vi "test.vi"() -> ()   [LabVIEW 2015]
uses:
  <vilib>/Analysis/6fits.llb/Curve Fitting Criteria.ctl
  APP/subject_class/elabPhases.ctl
  <userlib>/Read_Excel_Values.llb/GetXL_CellValues_2D_String.vi
  <vilib>/Analysis/NI_AALPro.lvlib
  APP/subject_class/subject.lvclass
panel:
  out "Array":i32[](array[numeric])
  out "XY Graph 3":cluster{i32[], "Best Linear Fit":dbl[]}[](graph)
  in  "Stop Button":bool
  out "XY Graph 2":cluster{"Best Linear Fit":dbl[], dbl[]}[](graph)
  out "output array":string[][](array[string])
  out "Array 3":i32[](array[numeric])
  out "Array 2":string[](array[string])
  in  "path":path
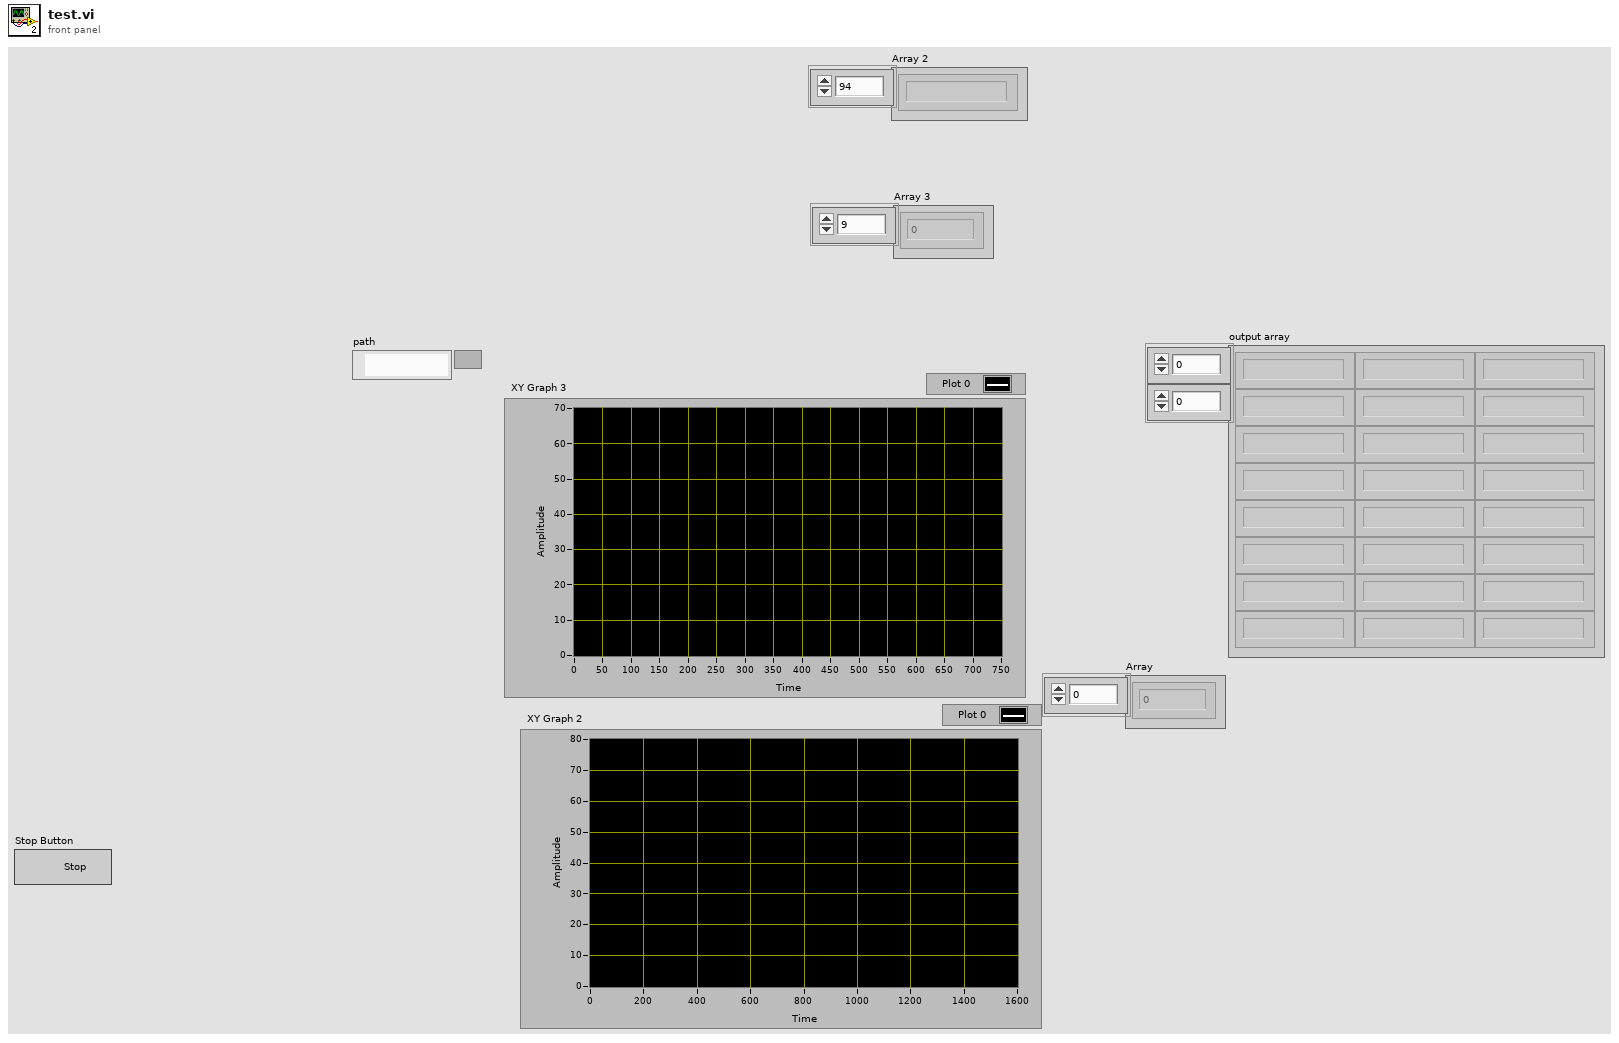
[diagram p1: front panel]
types:
  T1 = typedef "subject.lvclass/elabPhases.ctl" = enum16{"over", "under", "intersec"}
  T2 = typedef "NI_AALPro.lvlib/Curve Fitting Criteria.ctl" = u16
  T3 = cluster{"Excel._Application":refnum<k7>, "Workbooks":refnum<k7>}
  T4 = cluster{"Excel._Application":refnum<k7>, "Workbooks":refnum<k7>, "Open":refnum<k7>}
  T5 = cluster{"Excel._Application":refnum<k7>, "Workbooks":refnum<k7>, "Open":refnum<k7>, "Worksheets":refnum<k7>, "Excel._Worksheet":refnum<k7>}
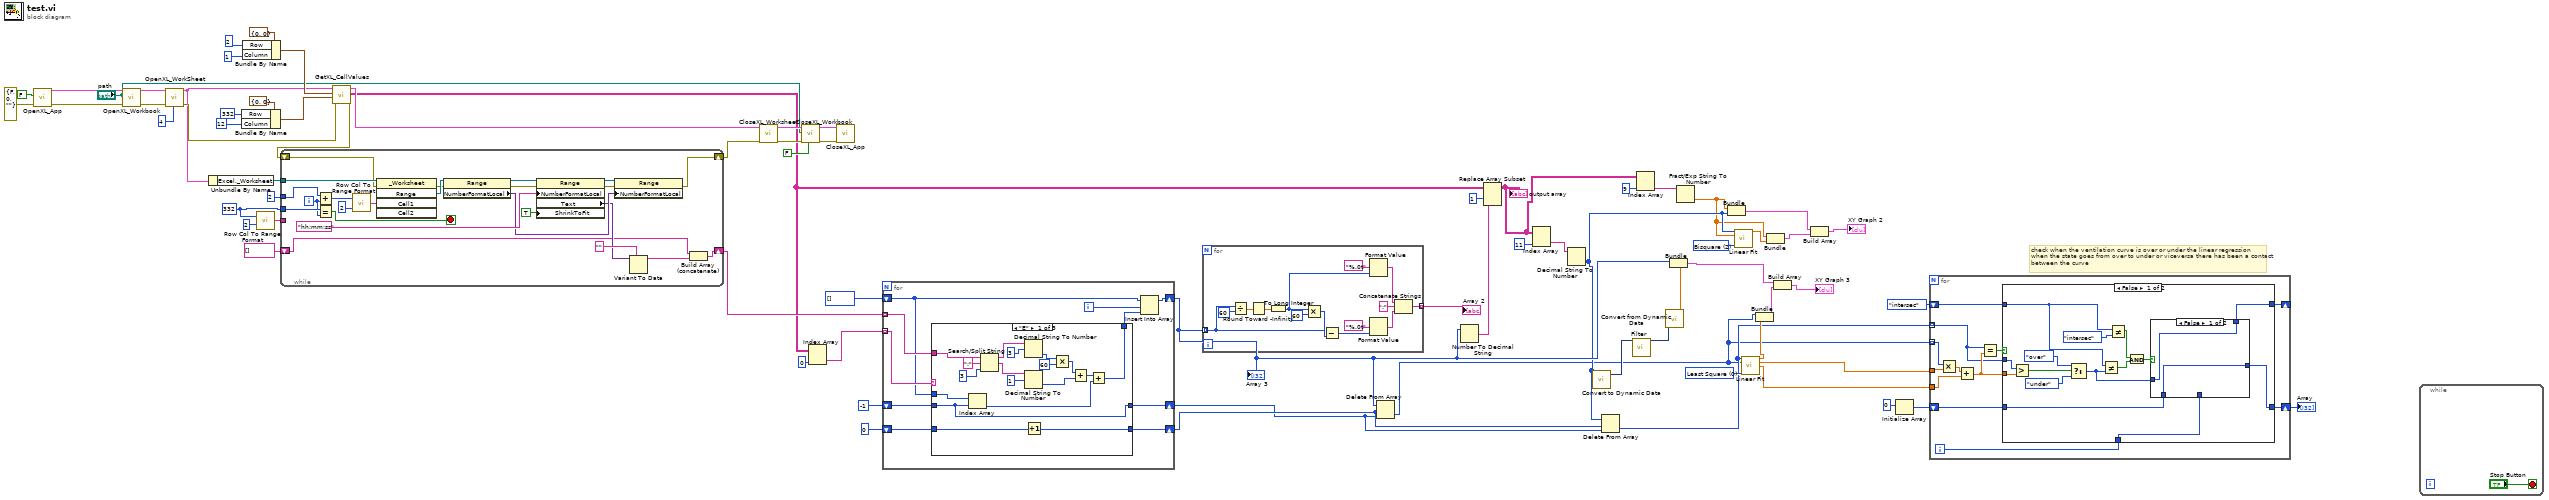
[diagram p0: block diagram]
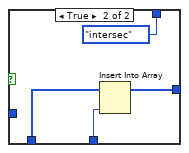
[diagram p2: hidden frame]
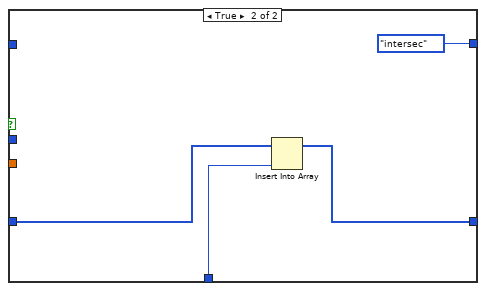
[diagram p3: hidden frame]
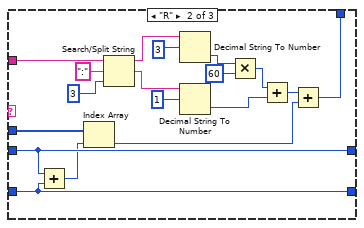
[diagram p4: hidden frame]
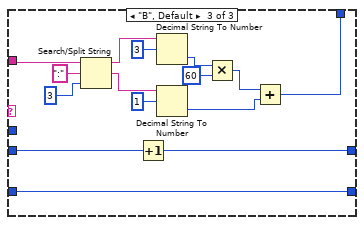
[diagram p5: hidden frame]
diagram:
  w9 = T2 2 items=["Least Square", "Least Absolute Residual", "Bisquare"] ("method")
  w32 = T2 0 items=["Least Square", "Least Absolute Residual", "Bisquare"] ("method")
  w42 = 332 ("Column")
  # "check when the ventilation curve is over or under the linear regression\nwhen the state goes from over to under or viceversa there has been a contact\nbetween the curve"
  n1 = call <userlib>:"OpenXL_App.vi"("error in (no error)"=errorcluster {"status"=FALSE, "code"=0, "source"=""}, "Visible"=FALSE) -> ("error out"=w66:errorcluster, "Refnum Cluster"=w67:T3)  [unwired: 8 in]
  n2 = call <userlib>:"OpenXL_Workbook.vi"("error in"=w66, "path"="path", "Refnum Cluster In"=w67) -> ("error out"=w65:errorcluster, "Refnum Cluster Out"=w47:T4)  [unwired: 7 in]
  n3 = call <userlib>:"OpenXL_WorkSheet.vi"("Sheet"=4, "error in (no error)"=w65, "Refnum Cluster In"=w47) -> ("error out"=w57:errorcluster, "Refnum Cluster Out"=w37:T5)  [unwired: 7 in]
  n4 = Unbundle By Name(w37) -> ("Excel._Worksheet"=w46:refnum<k7>)
  n5 = Bundle By Name(cluster=cluster{"Column":i32, "Row":i32} {"Column"=0, "Row"=0} ("Start"), "Row"=332, "Column"=12) -> (w58:cluster{"Column":i32, "Row":i32})
  n6 = Bundle By Name(cluster=cluster{"Column":i32, "Row":i32} {"Column"=0, "Row"=0} ("Start"), "Row"=2 ("Column"), "Column"=1) -> (w59:cluster{"Column":i32, "Row":i32})
  n7 = call <userlib>:"Row Col To Range Format.vi"("Column"=2, "Row"=w42) -> ("Output String"=w44:string)
  n8 = call-poly <userlib>:"GetXL_CellValues.vi"("error in"=w57, "End"=w58, "Start"=w59, "Refnum Cluster In"=w37) -> ("error out"=w40:errorcluster, "data"=w20:string[][], "Refnum Cluster Out"=w54:T5)  [unwired: 5 in]
  n9 = while {
    tunnel: w46 -> [w91]
    tunnel: w44 -> [_]
    shift-right: [w84] -> w38
    shift-left: string[] [] -> [w86]
    tunnel: w42 -> [w83]
    tunnel: 2 ("Column") -> [w79]
    shift-right: [w75] -> w39
    shift-left: w40 -> [w74]
    i -> [w78]
    stop <- w82 stop-if-true
    n10 = Add(x=w79, y=w78) -> (x+y=w77:i32)
    n11 = Equal?(x=w83, y=w78) -> (x = y?=w82:bool)
    n12 = call <userlib>:"Row Col To Range Format.vi"("Column"=2, "Row"=w77) -> ("Output String"=w80:string)
    n13 = invoke class="_Worksheet" method="Range"(reference=w91, error in=w74, "Cell1"=w80) -> (error out=w95:errorcluster, "Range"=w97:refnum<k7>)  [unwired: 2 in, 3 out]
    n14 = property class="Range"(reference=w97, error in=w95) -> (reference out=w96:refnum<k7>, error out=w94:errorcluster, "NumberFormatLocal"=w92:variant)
    n15 = property class="Range"(reference=w96, error in=w94, "NumberFormatLocal"="hh:mm:ss" ("data 3"), "ShrinkToFit"=TRUE) -> (reference out=w88:refnum<k7>, error out=w76:errorcluster, "Text"=w89:variant)
    n16 = property class="Range"(reference=w88, error in=w76, "NumberFormatLocal"=w92) -> (error out=w75:errorcluster)  [unwired: 1 out]
    n17 = Variant To Data(type="", Variant=w89) -> (data=w85:string)  [unwired: 1 in, 1 out]
    n18 = Build Array (concatenate)(w86, w85) -> (w84:string[])
  }
  n19 = call <userlib>:"CloseXL_Worksheet.vi"("error in (no error)"=w39, "Refnum Cluster In"=w54) -> ("error out"=w51:errorcluster, "Refnum Cluster Out"=w52:T4)  [unwired: 8 in]
  n20 = call <userlib>:"CloseXL_Workbook.vi"("Save? (F)"=FALSE, "error in (no error)"=w51, "path"="path", "Refnum Cluster In"=w52) -> ("error out"=w49:errorcluster, "Refnum Cluster Out"=w50:T3)  [unwired: 6 in]
  n21 = Index Array(array=w20, index (col)=0 ("disabled index (col)")) -> (element=w71:string[])  [unwired: 1 in]
  n22 = call <userlib>:"CloseXL_App.vi"("error in (no error)"=w49, "Refnum Cluster In"=w50) -> ()  [unwired: 9 in, 1 out]
  n23 = for {
    tunnel: w38 -> [w106] mode=indexing
    shift-right: [w105] -> w18
    shift-left: i32[] [] -> [w101]
    tunnel: w71 -> [w107] mode=indexing
    shift-right: [w102] -> w28
    shift-left: -1 -> [w99]
    shift-right: [w100] -> w29
    shift-left: 0 -> [w98]
    i -> [w104]
    n24 = case shown="\"E\"" w107 {
      tunnel: w106 -> [w117 w132 w158]
      tunnel: [w111 w131 w149] -> w103
      tunnel: w99 -> [w108 w127 w148]
      tunnel: [w108 w127 w147] -> w102
      tunnel: w101 -> [w115 w133 _]
      tunnel: w98 -> [w113 w128 w146]
      tunnel: [w112 w128 w146] -> w100
      frame "E" {
        n25 = Index Array(array=w115, index=w108) -> (element=w114:i32)
        n26 = Search/Split String(string=w117, search string/char (-)=":", offset (0)=3) -> (substring before match=w123:string, match + rest of string=w122:string)  [unwired: 1 out]
        n27 = Decimal String To Number(string=w123, offset=3) -> (number=w121:i32)  [unwired: 1 in, 1 out]
        n28 = Decimal String To Number(string=w122, offset=1) -> (number=w118:i32)  [unwired: 1 in, 1 out]
        n29 = Increment(x=w113) -> (x+1=w112:i32)
        n30 = Multiply(x=w121, y=60) -> (x*y=w119:i32)
        n31 = Add(x=w119, y=w118) -> (x+y=w116:i32)
        n32 = Add(x=w116, y=w114) -> (x+y=w111:i32)
      }
      frame "R" {
        n33 = Add(x=w127, y=w128) -> (x+y=w126:i32)
        n34 = Index Array(array=w133, index=w126) -> (element=w134:i32)
        n35 = Search/Split String(string=w132, search string/char (-)=":", offset (0)=3) -> (substring before match=w141:string, match + rest of string=w140:string)  [unwired: 1 out]
        n36 = Decimal String To Number(string=w141, offset=3) -> (number=w139:i32)  [unwired: 1 in, 1 out]
        n37 = Decimal String To Number(string=w140, offset=1) -> (number=w136:i32)  [unwired: 1 in, 1 out]
        n38 = Multiply(x=w139, y=60) -> (x*y=w137:i32)
        n39 = Add(x=w137, y=w136) -> (x+y=w135:i32)
        n40 = Add(x=w135, y=w134) -> (x+y=w131:i32)
      }
      frame "B", Default {
        n41 = Search/Split String(string=w158, search string/char (-)=":", offset (0)=3) -> (substring before match=w155:string, match + rest of string=w154:string)  [unwired: 1 out]
        n42 = Increment(x=w148) -> (x+1=w147:i32)
        n43 = Decimal String To Number(string=w155, offset=3) -> (number=w153:i32)  [unwired: 1 in, 1 out]
        n44 = Decimal String To Number(string=w154, offset=1) -> (number=w150:i32)  [unwired: 1 in, 1 out]
        n45 = Multiply(x=w153, y=60) -> (x*y=w151:i32)
        n46 = Add(x=w151, y=w150) -> (x+y=w149:i32)
      }
    }
    n47 = Insert Into Array(array=w101, index=w104, new element=w103) -> (w105:i32[])
  }
  "Array 3" <- w18
  n48 = for {
    tunnel: w18 -> [w168] mode=indexing
    tunnel: [w167] -> w13 mode=indexing
    n49 = Divide(x=w168, y=60) -> (x/y=w166:dbl)
    n50 = Round Toward -Infinity(1:w166) -> (0:w165:dbl)
    n51 = To Long Integer(number=w165) -> (32bit integer=w161:i32)
    n52 = Multiply(x=w161, y=60) -> (x*y=w169:i32)
    n53 = Subtract(x=w168, y=w169) -> (x-y=w163:i32)
    n54 = Format Value(format string="%.0t", value (0)=w161) -> (output string=w162:string)  [unwired: 1 in]
    n55 = Format Value(format string="%.0t", value (0)=w163) -> (output string=w159:string)  [unwired: 1 in]
    n56 = Concatenate Strings(w162, ":" ("string"), w159) -> (w167:string)
  }
  "Array 2" <- w13
  n57 = Delete From Array(array=w18, length=w29, index=w28) -> (deleted portion=w5:i32[])  [unwired: 1 out]
  n58 = Number To Decimal String(number=w18) -> (decimal integer string=w17:string[])  [unwired: 1 in]
  n59 = Replace Array Subset(array=w20, new element=w17, index (col)=1 ("disabled index (col)")) -> (w26:string[][])  [unwired: 1 in]
  "output array" <- w26
  n60 = Index Array(array=w26, index (col)=11 ("index (row)")) -> (element=w35:string[])  [unwired: 1 in]
  n61 = Decimal String To Number(string=w35) -> (number=w11:i32[])  [unwired: 2 in, 1 out]
  n62 = call "Convert to Dynamic Data"("Array"=w11) -> ("Dynamic Data Type"=w34:dynamicdata)  [unwired: 3 in]
  n63 = Delete From Array(array=w11, length=w29, index=w28) -> (deleted portion=w6:i32[])  [unwired: 1 out]
  n64 = call "Filter"("Signal"=w34) -> ("Filtered Signal"=w33:dynamicdata)  [unwired: 9 in, 1 out]
  n65 = Index Array(array=w26, index (col)=9 ("index (row)")) -> (element=w25:string[])  [unwired: 1 in]
  n66 = call "Convert from Dynamic Data"("Dynamic Data Type"=w33) -> ("Array"=w12:dbl[])  [unwired: 3 in]
  n67 = Bundle(w18, "Array"=w12) -> (w31:cluster{i32[], "Array":dbl[]})  [unwired: 1 in]
  n68 = Fract/Exp String To Number(string=w25) -> (number=w10:dbl[])  [unwired: 3 in, 1 out]
  n69 = Bundle(w10, w11) -> (w24:cluster{dbl[], i32[]})  [unwired: 1 in]
  n70 = call <vilib>:"Linear Fit.vi"("Y"=w11, "X"=w10, "method"=w9) -> ("Best Linear Fit"=w22:dbl[])  [unwired: 8 in, 4 out]
  n71 = call <vilib>:"Linear Fit.vi"("Y"=w6, "X"=w5, "method"=w32) -> ("Best Linear Fit"=w16:dbl[], "slope"=w7:dbl, "intercept"=w8:dbl)  [unwired: 8 in, 2 out]
  n72 = Bundle(w5, "Best Linear Fit"=w16) -> (w30:cluster{i32[], "Best Linear Fit":dbl[]})  [unwired: 1 in]
  n73 = Bundle(w10, "Best Linear Fit"=w22) -> (w23:cluster{dbl[], "Best Linear Fit":dbl[]})  [unwired: 1 in]
  n74 = Build Array(w31, w30) -> (→"XY Graph 3":cluster{i32[], "Best Linear Fit":dbl[]}[])
  n75 = Build Array(w24, w23) -> (→"XY Graph 2":cluster{dbl[], "Best Linear Fit":dbl[]}[])
  n76 = Initialize Array(0 ("element")) -> (w2:i32[])  [unwired: 1 in]
  n77 = for {
    tunnel: w8 -> [w181]
    tunnel: w7 -> [w184]
    tunnel: w6 -> [w174] mode=indexing
    tunnel: w5 -> [w183] mode=indexing
    shift-right: [w176] -> _
    shift-left: elabPhases."intersec" ("elabPhases") -> [w173]
    shift-right: [w178] -> w1
    shift-left: w2 -> [w179]
    i -> [w177]
    n78 = Multiply(x=w183, y=w184) -> (x*y=w182:dbl)
    n79 = Add(x=w182, y=w181) -> (x+y=w175:dbl)
    n80 = Equal?(x=w174, y=w175) -> (x = y?=w180:bool)
    n81 = case shown="False" w180 {
      tunnel: w179 -> [w191 w209]
      tunnel: [w189 w208] -> w178
      tunnel: w177 -> [w190 w207]
      tunnel: [w188 elabPhases."intersec" ("elabPhases")] -> w176
      tunnel: w175 -> [w199 _]
      tunnel: w174 -> [w198 _]
      tunnel: w173 -> [w186 _]
      frame False {
        n82 = Greater?(x=w198, y=w199) -> (0:w197:bool)
        n83 = Select(t=elabPhases."over" ("elabPhases"), s=w197, f=elabPhases."under" ("elabPhases")) -> (s? t:f=w185:T1)
        n84 = Not Equal?(x=w186, y=w185) -> (x != y?=w194:bool)
        n85 = Not Equal?(x=w186, y=elabPhases."intersec") -> (x != y?=w193:bool)
        n86 = And(x=w193, y=w194) -> (x .and. y?=w192:bool)
        n87 = case shown="False" w192 {
          tunnel: w191 -> [w201 w205]
          tunnel: w190 -> [_ w204]
          tunnel: [w201 w203] -> w189
          tunnel: [w200 elabPhases."intersec" ("y")] -> w188
          tunnel: w185 -> [w200 _]
          frame False {
          }
          frame True {
            n88 = Insert Into Array(array=w205, new element=w204) -> (w203:i32[])  [unwired: 1 in]
          }
        }
      }
      frame True {
        n89 = Insert Into Array(array=w209, new element=w207) -> (w208:i32[])  [unwired: 1 in]
      }
    }
  }
  "Array" <- w1
  n90 = while {
    stop <- "Stop Button" stop-if-true
  }
